vi "File.Change App Data folder to Local Tester Folder.vi"(11 "Sys":T1) -> (2 "AppDataDir":path, 3 "Sys Out":T1)   [LabVIEW 2018]
uses:
  <vilib>/KATE/Module/Module Sys Info.ctl
  <vilib>/KATE/Config/Stored Controls/Class.SaveCtrls.lvclass
  <vilib>/KATE/Event Log/Event Notification/Event Notification.lvclass
  <vilib>/KATE/Config/App Data/Class.AppData.lvclass
  <vilib>/KATE/Subscription/Subscription.lvclass
  <vilib>/KATE/Queues/Q.Element.ctl
  <vilib>/KATE/Module/Module.SW Version Info.ctl
  <vilib>/KATE/Module/Module Config.ctl
  <vilib>/KATE/Module/Module.Working Dirs.ctl
  <vilib>/KATE/Files/File Utils.lvlib
  <vilib>/KATE/Queues/Queue Utils.lvlib
  <vilib>/KATE/Module/Module Utils.lvlib
panel:
  # "Name, PN, Version, Note"
  # "Name, PN, Version, Note"
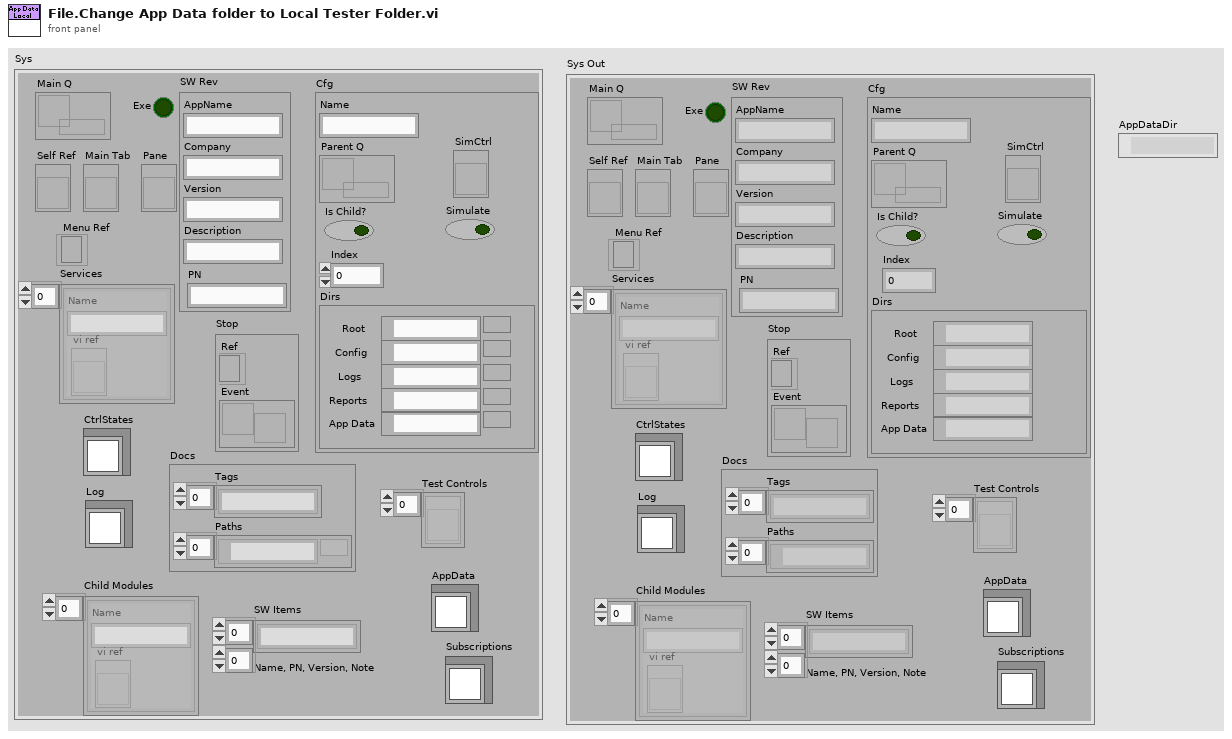
[diagram p1: front panel]
types:
  T1 = typedef "KATE_Lib.lvlib/Module Utils.lvlib/Module Sys Info.ctl" = cluster{"Main Q":refnum<queue>, "Exe":bool, "SW Rev":T2, "Self Ref":refnum<vi>, "Main Tab":refnum<vi>, "Pane":refnum<vi>, "Stop":cluster{"Ref":refnum<event-registration>, "Event":refnum<user-event>}, "Cfg":T3, "Services":cluster{"Name":string, "vi ref":refnum<vi>}[], "Menu Ref":refnum<k9>, "CtrlStates":refnum<class "Class.SaveCtrls.lvclass">, "Docs":cluster{"Tags":string[], "Paths":path[]}, "Log":refnum<class "Event Notification.lvclass">, "Test Controls":refnum<vi>[], "Child Modules":cluster{"Name":string, "vi ref":refnum<vi>}[], "SW Items":string[][], "AppData":refnum<class "Class.AppData.lvclass">, "Subscriptions":refnum<class "Subscription.lvclass">}
  T2 = typedef "KATE_Lib.lvlib/Module Utils.lvlib/Module.SW Version Info.ctl" = cluster{"AppName":string, "Company":string, "Version":string, "Description":string, "PN":string}
  T3 = typedef "KATE_Lib.lvlib/Module Utils.lvlib/Module Config.ctl" = cluster{"Name":string, "Parent Q":refnum<queue>, "Is Child?":bool, "Index":i32, "Dirs":T4, "Simulate":bool, "SimCtrl":refnum<vi>}
  T4 = typedef "KATE_Lib.lvlib/Module Utils.lvlib/Module.Working Dirs.ctl" = cluster{"Root":path, "Config":path, "Logs":path, "Reports":path, "App Data":path}
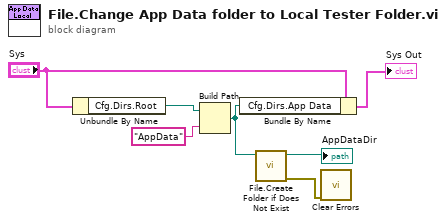
[diagram p0: block diagram]
diagram:
  n1 = Unbundle By Name("Sys") -> ("Cfg.Dirs.Root"=w6:path)
  n2 = Build Path(base path=w6, name or relative path="AppData") -> (appended path=w3:path)
  n3 = Bundle By Name(cluster="Sys", "Cfg.Dirs.App Data"=w3) -> (→"Sys Out":T1)
  n4 = call <vilib>:"File.Create Folder if Does Not Exist.vi"("Path"=w3) -> ("error out"=w1:errorcluster, "Dup Path"=→"AppDataDir":path)  [unwired: 8 in, 1 out]
  n5 = call <vilib>:"Clear Errors.vi"("error in (no error)"=w1) -> ()  [unwired: 5 in, 2 out]
